vi "SequenceAcquisitionSaveMultipleTiffImage.vi"() -> ()   [LabVIEW 2020]
uses:
  C:/Users/Public/Documents/Photometrics/PMQI-LabViewSamples/Examples/2018/Dependencies/PVCamNET.dll
  Dependencies/PVCamNET.dll
panel:
  out "SavingPath":string
  out "Boolean":bool
  in  "?":bool
  out "Capturing":bool
  in  "?":bool
  in  "FramesToCapture":u16
  in  "Exposure":u32
  in  "?":bool
  # "SequenceAcqusitionSaveMultipleTiffImage.vi\n\nDescription:\nThis sample code lets the user use sequence mode and save a TIFF image with \nthe user's preferred buffer size (framesToCapture) and exposure time. \n\nSteps to run:\n1. Go to Block Diagram and update SavingPath (Example: d:\\Temp\\ )\n2. Click \"Run\"\n3. Enter FramesToCapture and Exposure time\n4. Click \"START\"\n5. Click \"SAVE\"\n6. Click \"CLOSE\""
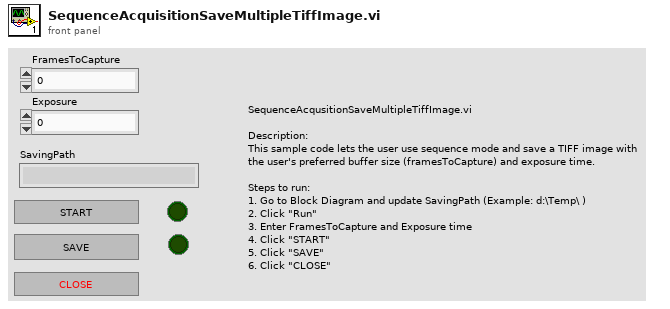
[diagram p1: front panel]
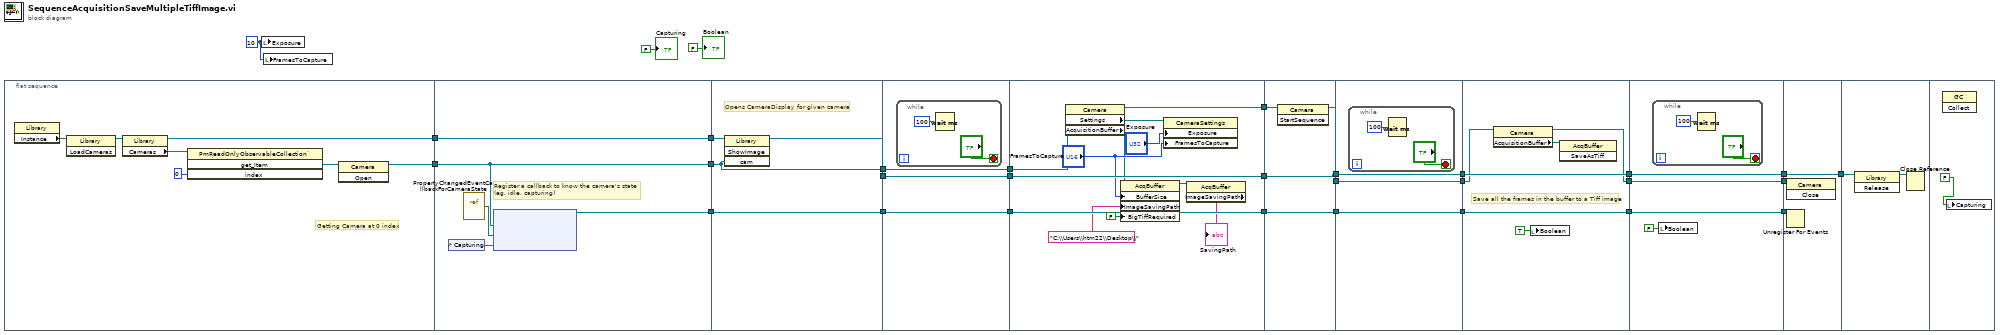
[diagram p0: block diagram]
diagram:
  w11 = u32 10 ("Exposure")
  n1 = flat-sequence {
    tunnel: [w33] -> w30
    tunnel: [w34] -> w29
    tunnel: w30 -> [w42]
    tunnel: [w42] -> w28
    tunnel: w29 -> [w39]
    tunnel: [w39] -> w27
    tunnel: [w38] -> w26
    tunnel: w28 -> [w46]
    tunnel: w27 -> [w45]
    tunnel: [w45] -> w24
    tunnel: [w44] -> w25
    tunnel: [w43] -> w23
    tunnel: w26 -> [w43]
    tunnel: w25 -> [w49]
    tunnel: [w49] -> w22
    tunnel: w24 -> [w48]
    tunnel: [w48] -> w21
    tunnel: [w47] -> w20
    tunnel: w23 -> [w47]
    tunnel: [w63] -> w19
    tunnel: [w62] -> w18
    tunnel: w22 -> [w62]
    tunnel: w21 -> [w61]
    tunnel: [w58] -> w17
    tunnel: w20 -> [w58]
    tunnel: w19 -> [w65]
    tunnel: [w64] -> w16
    tunnel: w18 -> [w67]
    tunnel: [w67] -> w15
    tunnel: [w66] -> w14
    tunnel: w17 -> [w66]
    tunnel: w16 -> [w70]
    tunnel: [w70] -> w10
    tunnel: w15 -> [w69]
    tunnel: [w69] -> w9
    tunnel: w14 -> [w68]
    tunnel: [w68] -> w8
    tunnel: w10 -> [w75]
    tunnel: [w74] -> w7
    tunnel: w9 -> [w78]
    tunnel: [w78] -> w5
    tunnel: w8 -> [w77]
    tunnel: [w77] -> w3
    tunnel: w7 -> [w82]
    tunnel: [w82] -> w6
    tunnel: w5 -> [w81]
    tunnel: [w81] -> w4
    tunnel: w3 -> [w80]
    tunnel: [w80] -> w2
    tunnel: w6 -> [w87]
    tunnel: w4 -> [w86]
    tunnel: [w86] -> w13
    tunnel: w2 -> [w85]
    tunnel: w13 -> [w89]
    frame #0 {
      # "Getting Camera at 0 index"
      n2 = property class="Library"() -> ("Instance"=w32:refnum<k24>)  [unwired: 2 in, 2 out]
      n3 = invoke class="Library" method="LoadCameras"(reference=w32) -> (reference out=w31:refnum<k24>)  [unwired: 2 in, 2 out]
      n4 = property class="Library"(reference=w31) -> (reference out=w33:refnum<k24>, "Cameras"=w37:refnum<k24>)  [unwired: 1 in, 1 out]
      n5 = invoke class="PmReadOnlyObservableCollection`" method="get_Item"(reference=w37, "index"=0) -> ("get_Item"=w35:refnum<k24>)  [unwired: 2 in, 3 out]
      n6 = invoke class="Camera" method="Open"(reference=w35) -> (reference out=w34:refnum<k24>)  [unwired: 2 in, 2 out]
    }
    frame #1 {
      # "Register a callback to know the camera's state \n(eg. idle, capturing)"
      n7 = control-ref of="Capturing"() -> (w41:refnum<vi>)
      n8 = vi-ref "PropertyChangedEventCallbackForCameraState.vi"() -> ("vi reference"=w40:refnum<vi>)
      n9 = node(w39, w40, w41) -> (w38:refnum<k27>)  [unwired: 2 in, 1 out]
    }
    frame #2 {
      # "Opens CameraDisplay for given camera"
      n10 = invoke class="Library" method="ShowImage"(reference=w46, "cam"=w45) -> (reference out=w44:refnum<k24>)  [unwired: 2 in, 3 out]
    }
    frame #3 {
      n11 = while {
        stop <- "?" stop-if-true
        n12 = Wait (ms)(milliseconds to wait=u32 100) -> ()  [unwired: 1 out]
      }
    }
    frame #4 {
      n13 = property class="Camera"(reference=w61) -> (reference out=w63:refnum<k24>, "Settings"=w60:refnum<k24>, "AcquisitionBuffer"=w56:refnum<k24>)  [unwired: 1 in, 1 out]
      n14 = property class="AcqBuffer"(reference=w56, "BufferSize"="FramesToCapture", "ImageSavingPath"="C:\\Users\\htm22\\Desktop\\" ("StreamSavingPath"), "BigTiffRequired"=FALSE) -> (reference out=w54:refnum<k24>)  [unwired: 1 in, 1 out]
      n15 = property class="CameraSettings"(reference=w60, "Exposure"="Exposure", "FramesToCapture"="FramesToCapture") -> ()  [unwired: 1 in, 2 out]
      n16 = property class="AcqBuffer"(reference=w54) -> ("ImageSavingPath"=→"SavingPath":string)  [unwired: 1 in, 2 out]
    }
    frame #5 {
      n17 = invoke class="Camera" method="StartSequence"(reference=w65) -> (reference out=w64:refnum<k24>)  [unwired: 2 in, 2 out]
    }
    frame #6 {
      n18 = while {
        stop <- "?" stop-if-true
        n19 = Wait (ms)(milliseconds to wait=u32 100) -> ()  [unwired: 1 out]
      }
    }
    frame #7 {
      # "Save all the frames in the buffer to a Tiff image"
      n20 = property class="Camera"(reference=w75) -> (reference out=w74:refnum<k24>, "AcquisitionBuffer"=w76:refnum<k24>)  [unwired: 1 in, 1 out]
      n21 = local write "Boolean"(TRUE ("Boolean")) -> ()
      n22 = invoke class="AcqBuffer" method="SaveAsTiff"(reference=w76) -> ()  [unwired: 2 in, 3 out]
    }
    frame #8 {
      n23 = while {
        stop <- "?" stop-if-true
        n24 = Wait (ms)(milliseconds to wait=u32 100) -> ()  [unwired: 1 out]
      }
      n25 = local write "Boolean"(FALSE ("Boolean")) -> ()
    }
    frame #9 {
      n26 = invoke class="Camera" method="Close"(reference=w87) -> ()  [unwired: 2 in, 3 out]
      n27 = Unregister For Events(event registration refnum=w85) -> ()  [unwired: 1 in, 1 out]
    }
    frame #10 {
      n28 = invoke class="Library" method="Release"(reference=w89) -> (reference out=w88:refnum<k24>)  [unwired: 2 in, 2 out]
      n29 = Close Reference(reference=w88) -> ()  [unwired: 1 in, 1 out]
    }
    frame #11 {
      n30 = invoke class="GC" method="Collect"() -> ()  [unwired: 3 in, 3 out]
      n31 = local write "Capturing"(FALSE ("Boolean")) -> ()
    }
  }
  n32 = local write "Exposure"(w11) -> ()
  n33 = local write "FramesToCapture"(w11) -> ()
  "Capturing" <- FALSE ("Capturing")
  "Boolean" <- FALSE ("Boolean")
